vi "nancheck.vi"(11 "nancheck_in":dbl) -> (3 "nancheck_out":dbl)   [LabVIEW 2011]
panel:
  # "Checks for NAN's and other numbers which can't be mathmatecally manipulated"
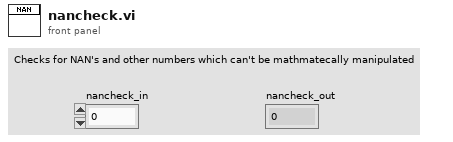
[diagram p1: front panel]
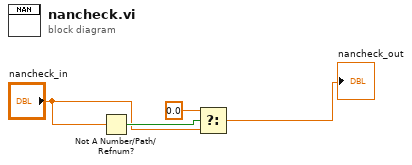
[diagram p0: block diagram]
diagram:
  n1 = Not A Number/Path/Refnum?(number/path/refnum="nancheck_in") -> (NaN/Path/Refnum?=w4:bool)
  n2 = Select(t=0.0, s=w4, f="nancheck_in") -> (s? t:f=→"nancheck_out":dbl)
